vi "Find LVLIBP Path.vi"(7 "Build Type":string, 10 "Files Generated by Build":path[](array[path])) -> (1 "Found ?":bool, 2 "Packed Library Path":path)   [LabVIEW 2020, in "LVLIBP CD XML Updater.lvlib"]
uses:
  LVLIBP CD XML Updater.lvlib
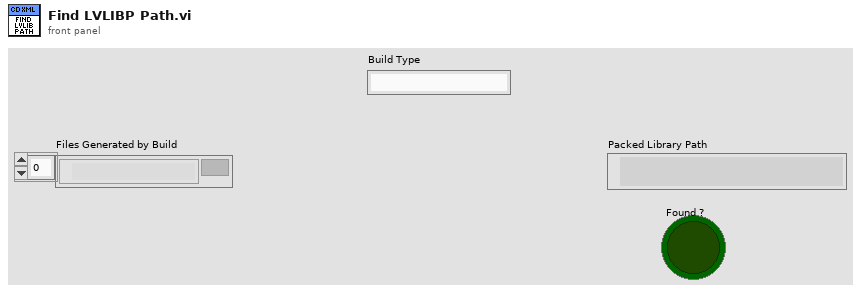
[diagram p1: front panel]
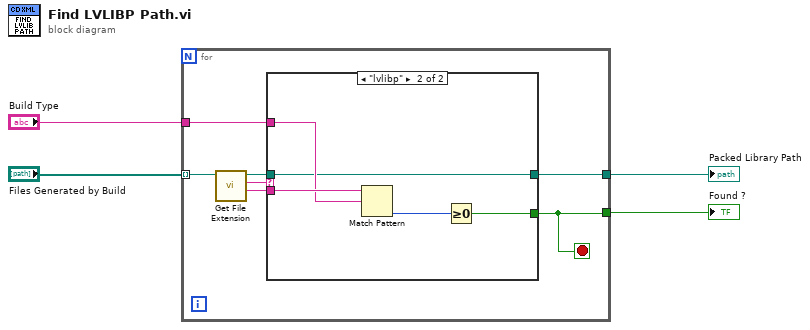
[diagram p0: block diagram]
diagram:
  n1 = for {
    tunnel: "Files Generated by Build" -> [w11] mode=indexing
    tunnel: "Build Type" -> [w8]
    tunnel: [w6] -> w1
    tunnel: [w5] -> w2
    stop <- w6 stop-if-true
    n2 = call <vilib>:"Get File Extension.vi"("file"=w11) -> ("filename without extension"=w9:string, "lowercase file extension"=w10:string, "dup file"=w7:path)  [unwired: 6 in, 2 out]
    n3 = case shown="\"lvlibp\"" w10 {
      tunnel: w9 -> [_ w16]
      tunnel: w8 -> [_ w15]
      tunnel: w7 -> [_ w12]
      tunnel: [_ w13] -> w6
      tunnel: [_ w12] -> w5
      frame "None", Default {
      }
      frame "lvlibp" {
        n4 = Match Pattern(string=w16, regular expression=w15) -> (offset past match=w14:i32)  [unwired: 1 in, 3 out]
        n5 = Greater Or Equal To 0?(x=w14) -> (x >= 0?=w13:bool)
      }
    }
  }
  "Packed Library Path" <- w2
  "Found ?" <- w1
